vi "Measurement Logic.vi"() -> ()   [LabVIEW 2024, in "NIDmmDcRmsMeasurement.lvlib"]
uses:
  NIDmmDCRmsMeasurement.lvlib
  <vilib>/MeasurementLink/MeasurementLink Measurement Server/Measure Call Context/Measure Call Context.lvclass
  Measurement Configuration.ctl
  Typedefs/Function.ctl
  Measurement Results.ctl
  <vilib>/MeasurementLink/MeasurementLink niDMM/Initialize Sessions - 1Sess.vi
  <instrlib>/niDMM/nidmm.llb/niDMM Read Waveform (waveform data).vi
  <vilib>/measure/madcrms.llb/Basic Averaged DC-RMS for 1 Chan.vi
  <vilib>/MeasurementLink/MeasurementLink niDMM/MeasurementLink niDMM.lvlib
  <vilib>/MeasurementLink/MeasurementLink Session Management V1/Session Reservation/Session Reservation.lvclass
  <vilib>/measure/NI_MAPro.lvlib
panel:
  out "measurement results":T1
  in  "measurement configuration":T2={"Range"=10.0, "Function"=1003, "Number of Samples"=1000.0, "Pin Name"="", "Sample Rate (Hz)"=1800000.0} {"Sample Rate (Hz)" format="%_2p"; "Number of Samples" format="%_1p"; "Function" items=["Waveform Voltage"=1003, "Waveform Current"=1004]}
  in  "error in":errorcluster
  out "error out":errorcluster
  out "measure call context out":refnum<class "Measure Call Context.lvclass">
  in  "measure call context in":refnum<class "Measure Call Context.lvclass">
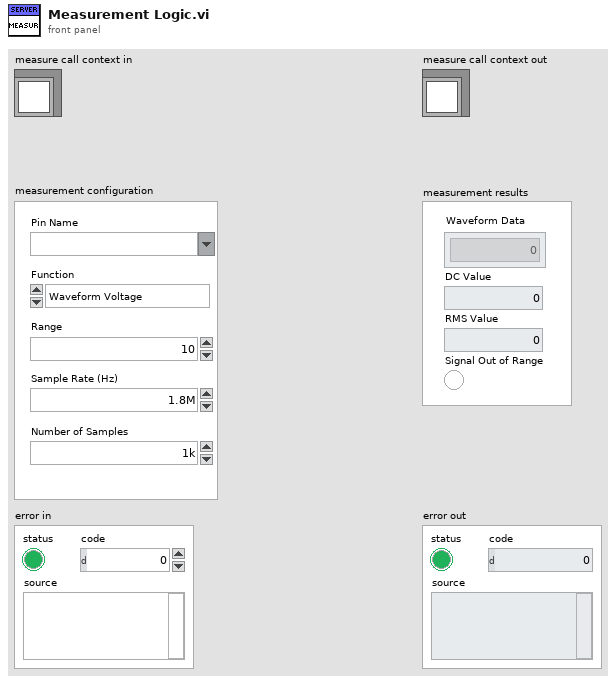
[diagram p1: front panel]
types:
  T1 = typedef "NIDmmDcRmsMeasurement.lvlib/Measurement Results.ctl" = cluster{"DC Value":dbl, "RMS Value":dbl, "Signal Out of Range":bool, "Waveform Data":dbl[]}
  T2 = typedef "NIDmmDcRmsMeasurement.lvlib/Measurement Configuration.ctl" = cluster{"Range":dbl, "Function":T3, "Number of Samples":dbl, "Pin Name":string, "Sample Rate (Hz)":dbl}
  T3 = typedef "NIDmmDcRmsMeasurement.lvlib/Function.ctl" = i32
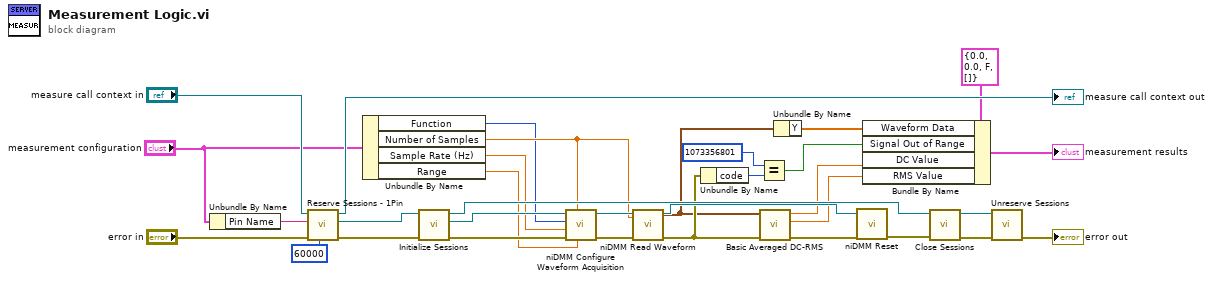
[diagram p0: block diagram]
diagram:
  n1 = Unbundle By Name("measurement configuration") -> ("Pin Name"=w33:string)
  n2 = call <vilib>:"Reserve Sessions - 1Pin.vi"("timeout (ms)"=60000, "error in"="error in", "pin or relay name"=w33, "measurement context in"="measure call context in") -> ("error out"=w14:errorcluster, "session reservation out"=w15:refnum<class "Session Reservation.lvclass">, "measurement context out"=→"measure call context out":refnum<class "Measure Call Context.lvclass">)  [unwired: 5 in]
  n3 = Unbundle By Name("measurement configuration") -> ("Function"=w16:T3, "Number of Samples"=w20:dbl, "Sample Rate (Hz)"=w17:dbl, "Range"=w18:dbl)
  n4 = call-poly <vilib>:"Initialize Sessions.vi"("error in"=w14, "session reservation in"=w15) -> ("error out"=w26:errorcluster, "session"=w27:refnum<k15>, "session reservation out"=w32:refnum<class "Session Reservation.lvclass">)  [unwired: 6 in, 1 out]
  n5 = call <instrlib>:"niDMM Configure Waveform Acquisition.vi"("Range"=w18, "Waveform Points"=w20, "error in (no error)"=w26, "Rate"=w17, "Function"=w16, "instrument handle"=w27) -> ("error out"=w25:errorcluster, "instrument handle out"=w24:refnum<k15>)  [unwired: 4 in]
  n6 = call-poly <instrlib>:"niDMM Read Waveform.vi"("Number To Read"=w20, "error in (no error)"=w25, "instrument handle"=w24) -> ("error out"=w5:errorcluster, "Waveform Data"=w3:waveform(dbl), "instrument handle out"=w10:refnum<k15>)  [unwired: 5 in, 1 out]
  n7 = Unbundle By Name(w5) -> ("code"=w23:i32)
  n8 = Equal?(x=1073356801 ("y"), y=w23) -> (x = y?=w21:bool)
  n9 = call-poly <vilib>:"Basic Averaged DC-RMS.vi"("error in (no error)"=w5, "signal in"=w3) -> ("error out"=w6:errorcluster, "RMS value"=w4:dbl, "DC value"=w2:dbl)  [unwired: 6 in, 1 out]
  n10 = Unbundle By Name(w3) -> ("Y"=w8:dbl[])
  n11 = call <instrlib>:"niDMM Reset.vi"("error in (no error)"=w6, "instrument handle"=w10) -> ("error out"=w7:errorcluster)  [unwired: 8 in, 1 out]
  n12 = Bundle By Name(cluster=T1 {"DC Value"=0.0, "RMS Value"=0.0, "Signal Out of Range"=FALSE, "Waveform Data"=[]} ("measurement results"), "Waveform Data"=w8, "Signal Out of Range"=w21, "DC Value"=w2, "RMS Value"=w4) -> (→"measurement results":T1)
  n13 = call <vilib>:"Close Sessions.vi"("error in"=w7, "session reservation in"=w32) -> ("error out"=w12:errorcluster, "session reservation out"=w11:refnum<class "Session Reservation.lvclass">)  [unwired: 8 in]
  n14 = call <vilib>:"Unreserve Sessions.vi"("error in"=w12, "session reservation in"=w11) -> ("error out"=→"error out":errorcluster)  [unwired: 9 in]
